vi "PH_Cont-601k_PSU.constructor.vi"(0 "name":string, 2 "data in":string, 5 "error in(no error)":errorcluster) -> (14 "i ref out":refnum<vi>, 16 "data out":string, 19 "error out":errorcluster)   [LabVIEW 2014, in "PH_Cont-601k_PSU.lvlib"]
doc: "This is the constructor of a class.\n\nLicense Agreement for this software:\n\nCopyright (C)\nGesellschaft für Schwerionenforschung, GSI\nPlanckstr. 1\n64291 Darmstadt\nGermany\n\nContact: D.Beck@gsi.de \n\nThis program is free software; you can redistribute it and/or modify it under the terms of the \nGNU General Public License as published by the Free Software Foundation; either version 2 of \nthe license, or (at your option) any later version.\n\nThis program is distributed in the hope that it will be useful, but WITHOUT ANY WARRANTY; \nwithout even the implied warranty of MERCHANTABILITY or FITNESS FOR A PARTICULAR PURPOSE. See the GNU General License for more details (http://www.gnu.org).\n\nGesellschaft für Schwerionenforschung, GSI\nPlanckstr. 1, 64291 Darmstadt, Germany\nFor all questions and ideas contact: M.Richter@gsi.de, H.Brand@gsi.de or D.Beck@gsi.de.\nLast update: 16-JUN-2004"
uses:
  PH_Cont-601k_PSU.lvlib
  PH_Cont-601k_PSU.Device Informaton.ctl
  CS_Core/CSSystem/CSSystemLib/CSSystemLib.lvlib
  PH_Basics/PH_Class/PH_Class.lvlib
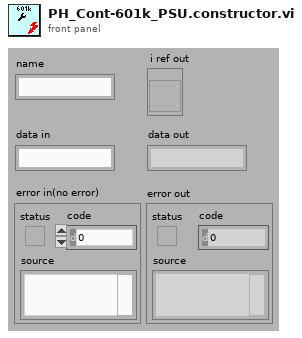
[diagram p1: front panel]
types:
  T1 = typedef "PH_Cont-601k_PSU.lvlib/PH_Cont-601k_PSU.Device Informaton.ctl" = cluster{"VISA resource":refnum<visa-resource-name>, "Driver Revision":string, "Firmware Revision":string}
  T2 = enum16{"SetAttribute", "GetAttribute", "CreateAttribute", "DestroyAttribute", "DestroyAllAtributes"}
  T3 = typedef "PH_Cont-601k_PSU.lvlib/PH_Cont-601k_PSU.i attribute.ctl" = cluster{"GUI Refs":T4, "Interlock":bool, "Service ID applied Voltage":i32, "Device Settings":cluster{"Configuration":T5, "Flash Interval [s]":dbl, "Mode":T6, "Voltage [V]":u16, "Charge":bool, "VISA resource name":refnum<visa-resource-name>}, "Readyness":T7, "Information":cluster{"VISA resource name":refnum<visa-resource-name>, "Tagname Power On":string, "Interlock":cluster{"Instance":string, "Tagname":string}, "Limits [V]":cluster{"Lower":dbl, "Upper":dbl}, "Tagname PSU On":string}, "R2S":bool, "Charge is allowed":bool}
  T4 = typedef "PH_Cont-601k_PSU.lvlib/PH_Cont-601k_PSU.GUI Refs.ctl" = cluster{"Power On":refnum<vi>, "Hard- and Software":refnum<vi>, "Device Status":refnum<vi>, "Device Error":refnum<vi>, "Configuration":refnum<vi>, "Flash Interval [s]":refnum<vi>, "Interlock":refnum<vi>, "Interlock Indicator":refnum<vi>, "Voltage [V]":refnum<vi>, "Readyness":refnum<vi>, "Mode":refnum<vi>, "Reset Error":refnum<vi>, "Expert working":refnum<vi>, "Charge":refnum<vi>, "PSU On":refnum<vi>}
  T5 = typedef "PH_Cont-601k_PSU.lvlib/PH_Cont-601k_PSU.Configuration.ctl" = u16
  T6 = typedef "PH_Cont-601k_PSU.lvlib/PH_Cont-601k_PSU.Mode.ctl" = enum32{"STOP", "STANDBY", "READY", "EMISSION", "ERROR"}
  T7 = typedef "PH_Cont-601k_PSU.lvlib/PH_Cont-601k_PSU.Readyness.ctl" = cluster{"Program":T8, "Device":T9}
  T8 = typedef "PH_Cont-601k_PSU.lvlib/PH_Cont-601k_PSU.Readyness Program.ctl" = enum32{"OFF", "POWER", "INTERLOCK"}
  T9 = typedef "PH_Cont-601k_PSU.lvlib/PH_Cont-601k_PSU.Readyness Device.ctl" = enum32{"OFF", "CONNECTING", "CONNECTED", "OPERATING", "EOC", "ERROR"}
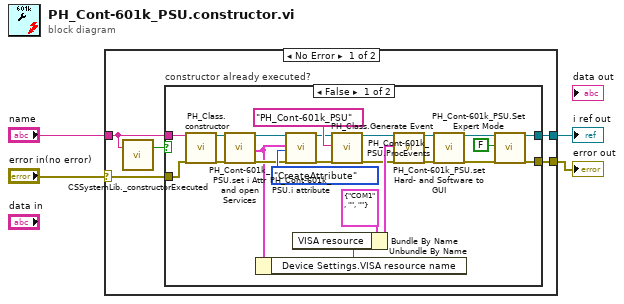
[diagram p0: block diagram]
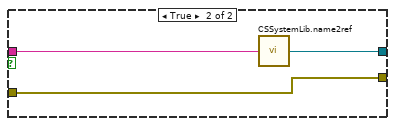
[diagram p2: hidden frame]
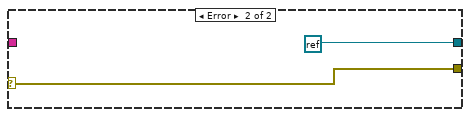
[diagram p3: hidden frame]
diagram:
  n1 = case shown="No Error" "error in(no error)" {
    selector: "error in(no error)" -> [w7 w36]
    tunnel: "name" -> [w6 _]
    tunnel: [w9 refnum<k0> refnum] -> w3
    tunnel: [w8 w36] -> w2
    frame No Error {
      n2 = call "CSSystemLib._constructorExecuted.vi"("name"=w6) -> ("constructor executed?"=w5:bool)  [unwired: 18 in]
      n3 = case "constructor already executed?" shown="False" w5 {
        tunnel: [w29 w34] -> w9
        tunnel: [w30 w33] -> w8
        tunnel: w7 -> [w15 w33]
        tunnel: w6 -> [w31 w35]
        frame False {
          n4 = call "PH_Class.constructor.vi"("name"=w31, "error in"=w15) -> ("i ref out"=w12:refnum<vi>, "error out"=w13:errorcluster)  [unwired: 15 in, 1 out]
          n5 = call "PH_Cont-601k_PSU.set i Attr and open Services.vi"("i ref in"=w12, "error in"=w13) -> ("i ref out"=w11:refnum<vi>, "i Attributes"=w14:T3, "error out"=w18:errorcluster)  [unwired: 15 in]
          n6 = Unbundle By Name(w14) -> ("Device Settings.VISA resource name"=w23:refnum<visa-resource-name>)
          n7 = call "PH_Cont-601k_PSU.i attribute.vi"("VI Refnum"=w11, "CLASS.i attribute"=w14, "Action"=T2."CreateAttribute", "error in (no error)"=w18) -> ("VI Refnum out"=w10:refnum<vi>, "error out"=w22:errorcluster)  [unwired: 13 in, 1 out]
          n8 = Bundle By Name(cluster=T1 {"VISA resource"="COM1", "Driver Revision"="", "Firmware Revision"=""} ("Hard- and Software"), "VISA resource"=w23) -> (w24:T1)
          n9 = call "PH_Class.Generate Event.vi"("i ref in"=w10, "Class"="PH_Cont-601k_PSU", "error in (no error)"=w22) -> ("i ref out"=w21:refnum<vi>, "error out"=w20:errorcluster)  [unwired: 15 in]
          n10 = call "PH_Cont-601k_PSU.set Hard- and Software to GUI.vi"("VI in"=w21, "Hard- and Software"=w24, "error in (no error)"=w20) -> ("VI out"=w16:refnum<vi>, "error out"=w17:errorcluster)  [unwired: 15 in]
          n11 = call "PH_Cont-601k_PSU.ProcEvents.vi"("i ref in"=w16, "error in"=w17) -> ("i ref out"=w27:refnum<vi>, "error out"=w26:errorcluster)  [unwired: 16 in]
          n12 = call "PH_Cont-601k_PSU.Set Expert Mode.vi"("VI in"=w27, "Expert working"=FALSE, "error in (no error)"=w26) -> ("VI out"=w29:refnum<vi>, "error out"=w30:errorcluster)  [unwired: 15 in]
        }
        frame True {
          n13 = call "CSSystemLib.name2ref.vi"("name"=w35) -> ("obj refnum"=w34:refnum<vi>)
        }
      }
    }
    frame Error {
    }
  }
  "i ref out" <- w3
  "error out" <- w2
